vi "Timer.vi"(8 "error in (no error)":errorcluster, 9 "Reset?":bool, 10 "Advance?":bool, 11 "Target Time":dbl) -> (0 "error out":errorcluster, 1 "Time Remaining":dbl, 2 "Done?":bool, 3 "Elapsed Time":dbl)   [LabVIEW 2026]
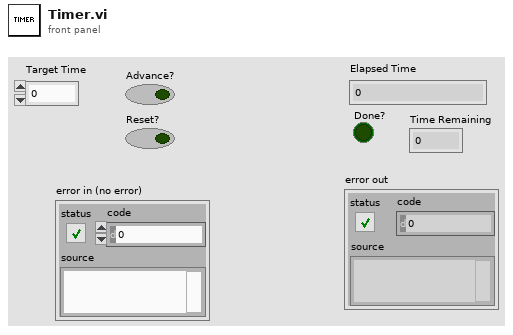
[diagram p1: front panel]
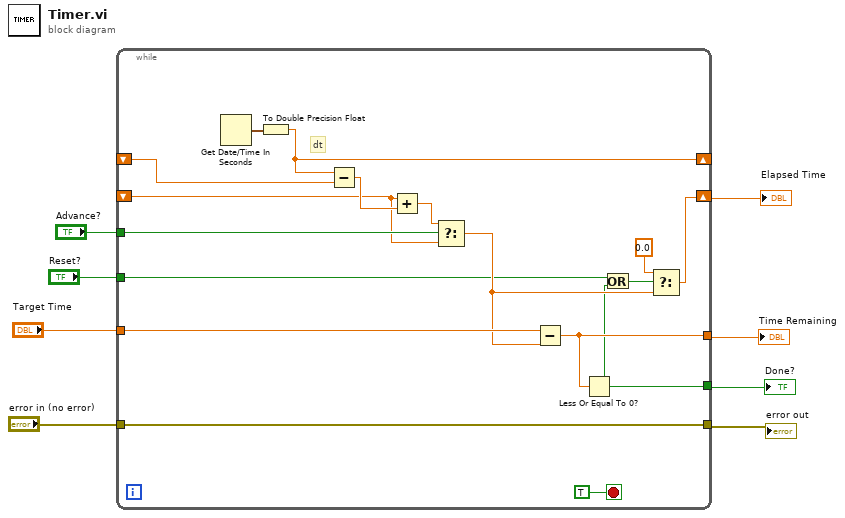
[diagram p0: block diagram]
diagram:
  n1 = while {
    shift-right: [w24] -> _
    shift-left: _ -> [w20]
    tunnel: "Reset?" -> [w9]
    tunnel: "error in (no error)" -> [w21]
    tunnel: [w21] -> w6
    tunnel: [w11] -> w5
    tunnel: "Advance?" -> [w17]
    shift-right: [w18] -> w4
    shift-left: _ -> [w13]
    tunnel: "Target Time" -> [w15]
    tunnel: [w12] -> w1
    stop <- TRUE stop-if-true
    # "dt"
    n2 = Get Date/Time In Seconds() -> (seconds since 1Jan1904=w23:timestamp)
    n3 = To Double Precision Float(number=w23) -> (double precision float=w24:dbl)
    n4 = Subtract(x=w24, y=w20) -> (x-y=w19:dbl)
    n5 = Add(x=w13, y=w19) -> (x+y=w16:dbl)
    n6 = Select(t=w16, s=w17, f=w13) -> (s? t:f=w14:dbl)
    n7 = Subtract(x=w15, y=w14) -> (x-y=w12:dbl)
    n8 = Less Or Equal To 0?(x=w12) -> (x <= 0?=w11:bool)
    n9 = Or(x=w9, y=w11) -> (x .or. y?=w10:bool)
    n10 = Select(t=0.0, s=w10, f=w14) -> (s? t:f=w18:dbl)
  }
  "Elapsed Time" <- w4
  "error out" <- w6
  "Done?" <- w5
  "Time Remaining" <- w1
